vi "Format Into Vector Statement.vi"(0 "Timeset (RFFE)":string="RFFE", 5 "CLK (1)":string="1", 7 "DATA (0)":string="0", 9 "Comment":string, 11 "error in (no error)":errorcluster, 12 "Label":string, 13 "Opcode":string) -> (4 "Vector Statement":string, 15 "error out":errorcluster)   [LabVIEW 2018, in "MIPI RFFE API.lvlib"]
uses:
  MIPI RFFE API.lvlib
  <vilib>/Utility/error.llb/whitespace.ctl
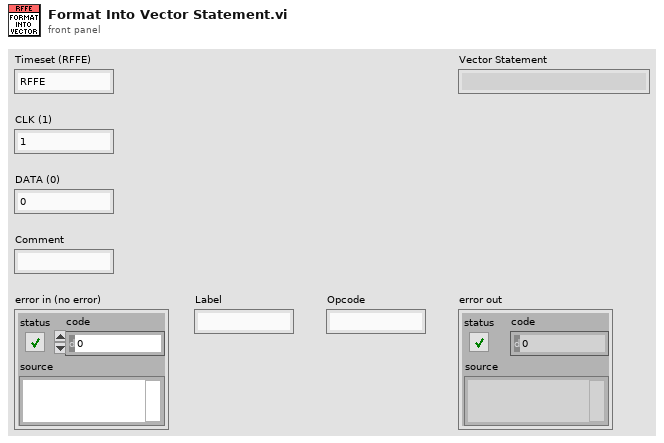
[diagram p1: front panel]
types:
  T1 = typedef "whitespace.ctl" = u16
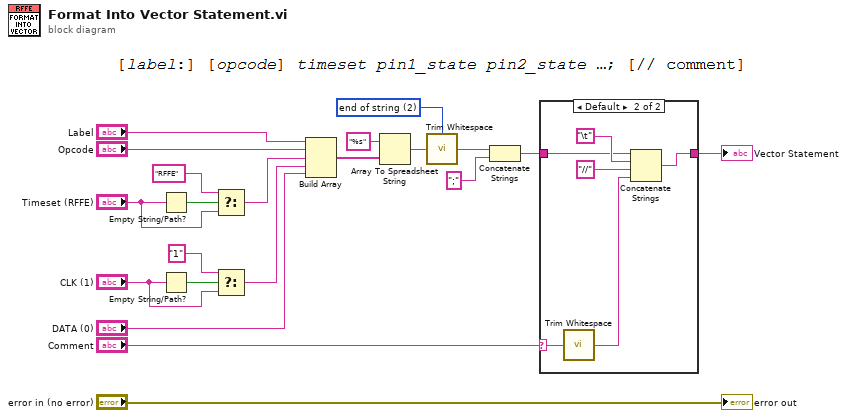
[diagram p0: block diagram]
diagram:
  w12 = T1 2 items=["both", "start of string", "end of string"] ("location (both)")
  n1 = Empty String/Path?(string/path="Timeset (RFFE)") -> (empty?=w8:bool)
  n2 = Empty String/Path?(string/path="CLK (1)") -> (empty?=w3:bool)
  n3 = Select(t="RFFE", s=w8, f="Timeset (RFFE)") -> (s? t:f=w5:string)
  n4 = Select(t="1", s=w3, f="CLK (1)") -> (s? t:f=w2:string)
  n5 = Build Array("Label", "Opcode", w5, w2, "DATA (0)") -> (w15:string[])
  n6 = Array To Spreadsheet String(array=w15, 3:"%s" ("format string")) -> (spreadsheet string=w13:string)  [unwired: 1 in]
  n7 = call <vilib>:"Trim Whitespace.vi"("string"=w13, "location (both)"=w12) -> ("trimmed string"=w11:string)
  n8 = Concatenate Strings(w11, ";" ("string")) -> (w9:string)
  n9 = case shown="Default" "Comment" {
    selector: "Comment" -> [_ w28]
    tunnel: [w22 w27] -> w17
    tunnel: w9 -> [w22 w23]
    frame "" {
    }
    frame Default {
      n10 = call <vilib>:"Trim Whitespace.vi"("string"=w28) -> ("trimmed string"=w24:string)  [unwired: 1 in]
      n11 = Concatenate Strings(w23, "\t", "//" ("string"), w24) -> (w27:string)
    }
  }
  "Vector Statement" <- w17
  "error out" <- "error in (no error)"
